vi "_fromString.vi"(8 "error in (no error)":errorcluster, 10 "<JSON>":string, 11 "CalibReport in":refnum<class "CalibReport.lvclass">) -> (0 "error out":errorcluster, 3 "CalibReport out":refnum<class "CalibReport.lvclass">)   [LabVIEW 2024, in "CalibReport.lvclass"]
uses:
  CalibReport.lvclass
  cReportEntry.ctl
  CalibReport.lvclass/CalibReport.ctl
  c4f6845c-cfdf-49d8-a0a9-c26fbf0a2c9f.vi
  6322d839-194b-485d-ae17-9a352b41fab0.vi
  698cc6d7-b9ca-4a3d-9f9c-ffbff705d8ab.vi
  <vilib>/JDP Science/JSONtext/Next JSON Value.vi
  <vilib>/JDP Science/JSONtext/String Subset.vi
  <vilib>/JDP Science/JSONtext/Parsing/Advance past next JSON Value (inlined COPY).vi
  <vilib>/JDP Science/JSONtext/Parsing/Advance past whitespace.vi
  <vilib>/JDP Science/JSONtext/Parsing/Advance past String.vi
  <vilib>/JDP Science/JSONtext/Parsing/Advance past Number.vi
  <vilib>/JDP Science/JSONtext/Parsing/Advance past Line Ending.vi
  <vilib>/JDP Science/JSONtext/Parsing/Parse Full Path or Item Name.vi
  <vilib>/JDP Science/JSONtext/Parsing/Advance past Array.vi
  <vilib>/JDP Science/JSONtext/Parsing/Advance past Object.vi
  <vilib>/JDP Science/JSONtext/support/Error Cluster From Code.vi
  <vilib>/JDP Science/JSONtext/Offset/Find Item Locations by Path.vi
  <vilib>/JDP Science/JSONtext/JSON text to Variant.vi
  <vilib>/JDP Science/JSONtext/LVClass Serializer/JSONtext LVClass Serializer.lvclass
  <vilib>/JDP Science/JSONtext/JSONtext.lvlib
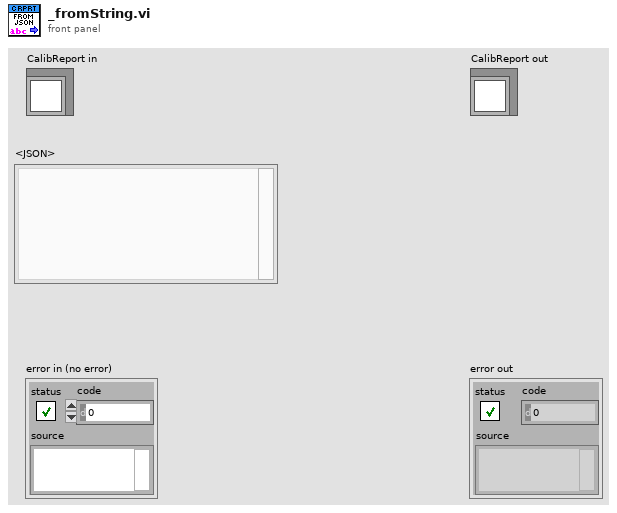
[diagram p1: front panel]
types:
  T1 = typedef "cReportEntry.ctl" = cluster{"Reference [kg]":dbl, "DUT value [kg]":dbl}
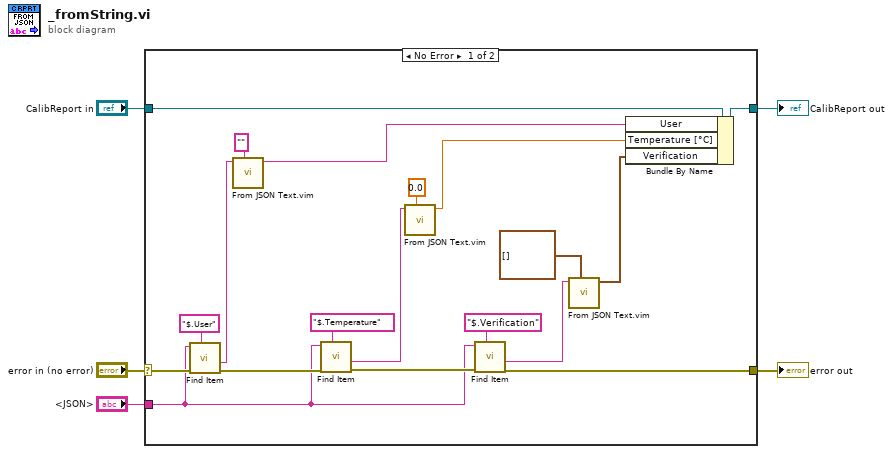
[diagram p0: block diagram]
diagram:
  n1 = case shown="No Error" "error in (no error)" {
    selector: "error in (no error)" -> [w23 w26]
    tunnel: [w10 w26] -> w4
    tunnel: [w9 w25] -> w2
    tunnel: "CalibReport in" -> [w24 w25]
    tunnel: "<JSON>" -> [w17 _]
    frame No Error {
      n2 = call <vilib>:"Find Item.vi"("$Path or Item Name"="$.User" ("String"), "error in (no error)"=w23, "JSON"=w17) -> ("error out"=w19:errorcluster, "<JSON>"=w15:string)  [unwired: 5 in, 2 out]
      n3 = call "From JSON Text.vim"("Data Type and Default Value"="" ("User"), "JSON"=w15) -> ("Data out"=w6:string)  [unwired: 8 in, 1 out]
      n4 = call <vilib>:"Find Item.vi"("$Path or Item Name"="$.Temperature" ("String"), "error in (no error)"=w19, "JSON"=w17) -> ("error out"=w18:errorcluster, "<JSON>"=w13:string)  [unwired: 5 in, 2 out]
      n5 = call "From JSON Text.vim"("Data Type and Default Value"=0.0 ("Temperature [°C]"), "JSON"=w13) -> ("Data out"=w7:dbl)  [unwired: 8 in, 1 out]
      n6 = call <vilib>:"Find Item.vi"("$Path or Item Name"="$.Verification" ("String"), "error in (no error)"=w18, "JSON"=w17) -> ("error out"=w10:errorcluster, "<JSON>"=w11:string)  [unwired: 5 in, 2 out]
      n7 = call "From JSON Text.vim"("Data Type and Default Value"=T1[] [] ("Verification"), "JSON"=w11) -> ("Data out"=w8:T1[])  [unwired: 8 in, 1 out]
      n8 = Bundle By Name(cluster=w24, "User"=w6, "Temperature [°C]"=w7, "Verification"=w8) -> (w9:refnum<class "CalibReport.lvclass">)
    }
    frame Error {
    }
  }
  "error out" <- w4
  "CalibReport out" <- w2
